vi "generate outputs.vi"(11 "output data":T1[](array[typedef])) -> (3 "data array w/o header":u32[](array[numeric]))   [LabVIEW 2013]
uses:
  profibus master action.ctl
  dynamic profibus.lvlib
  dataset.ctl
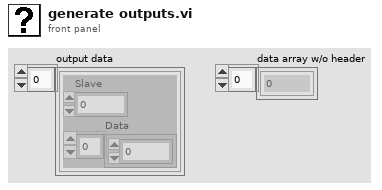
[diagram p1: front panel]
types:
  T1 = typedef "dynamic profibus.lvlib/dataset.ctl" = cluster{"Slave":u8, "Data":u8[]}
  T2 = typedef "dynamic profibus.lvlib/profibus master action.ctl" = enum8{"initialize", "uninitialize", "stop", "get input", "get input size", "set output", "get output size", "get diagnostic", "transfer data", "transfer diagnostics", "read many inputs"}
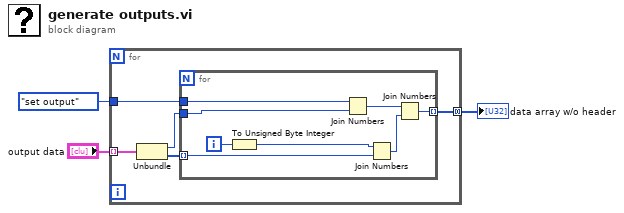
[diagram p0: block diagram]
diagram:
  n1 = for {
    tunnel: "output data" -> [w8] mode=indexing
    tunnel: profibus_master_action."set output" ("action") -> [w5]
    tunnel: [w4] -> w3 mode=concatenating
    n2 = Unbundle(w8) -> ("Slave"=w6:u8, "Data"=w7:u8[])
    n3 = for {
      tunnel: w7 -> [w12] mode=indexing
      tunnel: w6 -> [w10]
      tunnel: w5 -> [w13]
      tunnel: [w9] -> w4 mode=indexing
      i -> [w16]
      n4 = To Unsigned Byte Integer(number=w16) -> (unsigned 8bit integer=w11:u8)
      n5 = Join Numbers(hi=w13, lo=w10) -> ((hi.lo)=w14:u16)
      n6 = Join Numbers(hi=w11, lo=w12) -> ((hi.lo)=w15:u16)
      n7 = Join Numbers(hi=w14, lo=w15) -> ((hi.lo)=w9:u32)
    }
  }
  "data array w/o header" <- w3
